vi "LVClass_ModalCoef ctor From File.vi"(0 "ModalCoef in":refnum<class "ModalCoef.lvclass">, 7 "coefs_file_path":path, 11 "error in (no error)":errorcluster) -> (4 "ModalCoef out":refnum<class "ModalCoef.lvclass">, 8 "Comments":string, 15 "error out":errorcluster)   [LabVIEW 2020, in "ModalCoef.lvclass"]
doc: "ModalCoef constructor.\n\n--------------------------------------------------------------------------------\n\n<B>ModalCoefIn </B> : Constant Pointer to ModalCoef object.\n<B>ModalCoefOut </B> : Constant Pointer to ModalCoef object.\n<B>TypePhase </B> : TypePhase Phase mode reconstruction.\n<B>ErrorIn </B> : Error\n<B>ErrorOut </B> : Error\n\n--------------------------------------------------------------------------------"
uses:
  ModalCoef.lvclass
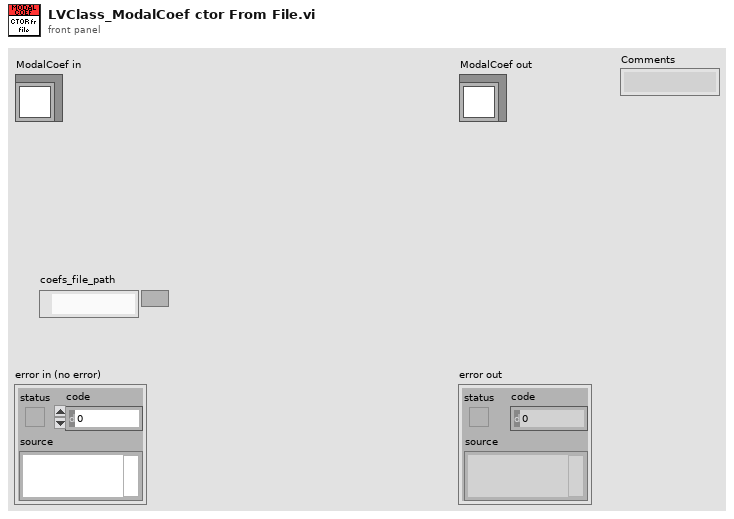
[diagram p1: front panel]
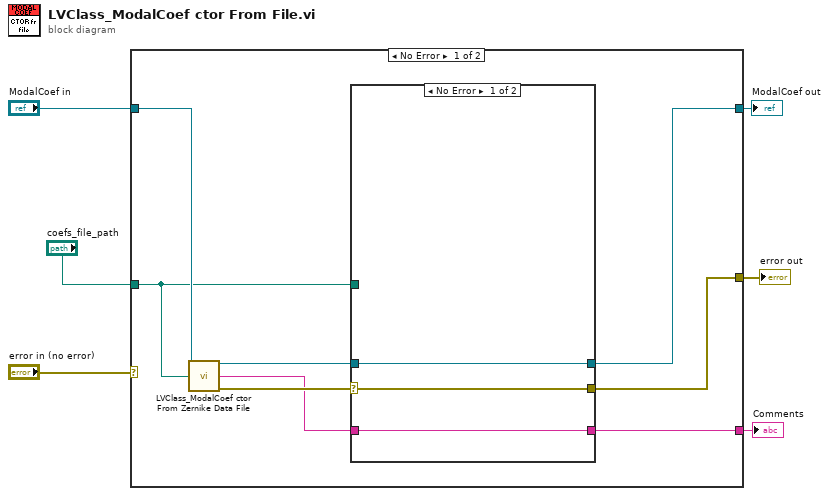
[diagram p0: block diagram]
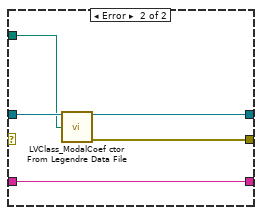
[diagram p2: hidden frame]
diagram:
  n1 = case shown="No Error" "error in (no error)" {
    selector: "error in (no error)" -> [_ w24]
    tunnel: [w10 w24] -> w5
    tunnel: [w12 w23] -> w3
    tunnel: "ModalCoef in" -> [w14 w23]
    tunnel: "coefs_file_path" -> [w9 _]
    tunnel: [w7 _] -> w1
    frame No Error {
      n2 = call "LVClass_ModalCoef ctor From Zernike Data File.vi"("ModalCoef (const)"=w14, "coefs_file_path"=w9) -> ("ModalCoef (new)"=w13:refnum<class "ModalCoef.lvclass">, "Comments"=w8:string, "error out"=w11:errorcluster)  [unwired: 11 in]
      n3 = case shown="No Error" w11 {
        selector: w11 -> [w16 _]
        tunnel: w13 -> [w17 w22]
        tunnel: [w17 w21] -> w12
        tunnel: [w16 w19] -> w10
        tunnel: w9 -> [_ w20]
        tunnel: w8 -> [w15 w18]
        tunnel: [w15 w18] -> w7
        frame No Error {
        }
        frame Error {
          n4 = call "LVClass_ModalCoef ctor From Legendre Data File.vi"("ModalCoef (const)"=w22, "coefs_file_path"=w20) -> ("ModalCoef (new)"=w21:refnum<class "ModalCoef.lvclass">, "error out"=w19:errorcluster)  [unwired: 11 in, 1 out]
        }
      }
    }
    frame Error {
    }
  }
  "error out" <- w5
  "ModalCoef out" <- w3
  "Comments" <- w1
